vi "Connect.vi"(8 "error in (no error)":errorcluster, 11 "MSOX6004 in":refnum<class "MSOX6004.lvclass">) -> (0 "error out":errorcluster, 3 "MSOX6004 out":refnum<class "MSOX6004.lvclass">)   [LabVIEW 2018, in "MSOX6004.lvlib" / "MSOX6004.lvclass"]
doc: "This Override method is used initiative the communication session with the Oscope instrument."
uses:
  MSOX6004.lvclass
  MSOX6004.lvclass/MSOX6004.ctl
  PPLs/Oscilloscope/Parent/Oscilloscope.lvlibp/Oscilloscope.lvclass
  <instrlib>/Keysight InfiniiVision/Keysight InfiniiVision.lvlib
  C:/Projects/LabVIEW/PPLs/Oscilloscope/Parent/Oscilloscope.lvlibp/Oscilloscope.lvclass
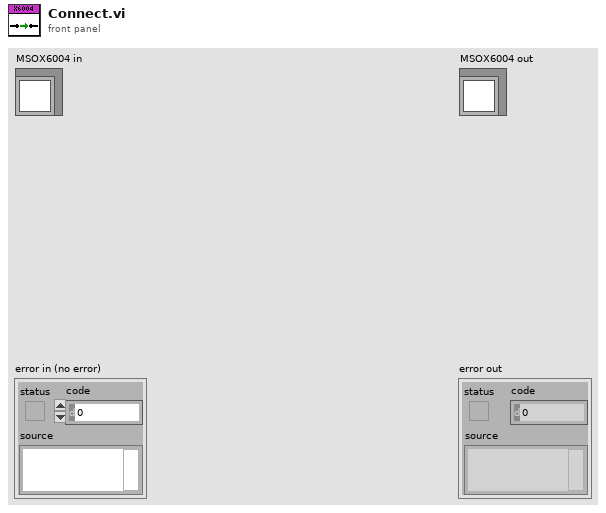
[diagram p1: front panel]
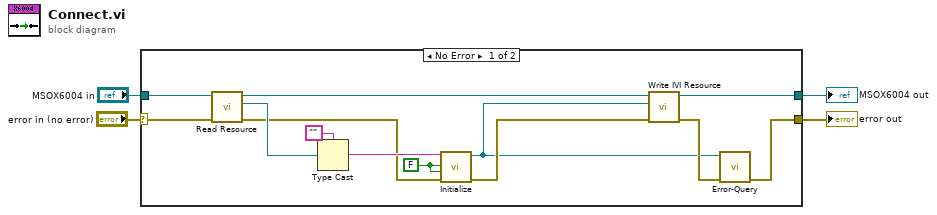
[diagram p0: block diagram]
diagram:
  n1 = case shown="No Error" "error in (no error)" {
    selector: "error in (no error)" -> [w16 w18]
    tunnel: "MSOX6004 in" -> [w17 w19]
    tunnel: [w7 w18] -> w2
    tunnel: [w6 w19] -> w1
    frame No Error {
      w12 = FALSE
      n2 = call "Read Resource.vi"("error in (no error)"=w16, "Oscilloscope in"=w17) -> ("error out"=w11:errorcluster, "Resource"=w15:refnum<visa-resource-name>, "Oscilloscope out"=w9:refnum<class "MSOX6004.lvclass">)  [unwired: 7 in]
      n3 = Type Cast(type="", x=w15) -> (*(type *) &x=w13:string)
      n4 = call <instrlib>:"Initialize.vi"("error in (no error)"=w11, "reset device (Off)"=w12, "id query (Off)"=w12, "resource string"=w13) -> ("error out"=w10:errorcluster, "instrument handle out"=w5:refnum<k15>)  [unwired: 6 in]
      n5 = call "Write IVI Resource.vi"("error in (no error)"=w10, "IVI Resource"=w5, "MSOX6004 in"=w9) -> ("error out"=w8:errorcluster, "MSOX6004 out"=w6:refnum<class "MSOX6004.lvclass">)  [unwired: 7 in]
      n6 = call <instrlib>:"Error-Query.vi"("error in (no error)"=w8, "instrument handle"=w5) -> ("error out"=w7:errorcluster)  [unwired: 6 in, 3 out]
    }
    frame Error {
    }
  }
  "error out" <- w2
  "MSOX6004 out" <- w1
